vi "getParameters.vi"(11 "AbortLowerM1M3Command in":refnum<class "AbortLowerM1M3Command.lvclass">) -> (2 "Parameters":T1, 3 "AbortLowerM1M3Command out":refnum<class "AbortLowerM1M3Command.lvclass">)   [LabVIEW 2016, in "AbortLowerM1M3Command.lvclass"]
uses:
  AbortLowerM1M3Command.lvclass
  DataTypes/Topics/CommandAbortLowerM1M3.ctl
  DataTypes/Topics/Parts/CommandId.ctl
  AbortLowerM1M3Command.lvclass/AbortLowerM1M3Command.ctl
  DataTypes/Topics/M1M3SupportTopics.lvlib
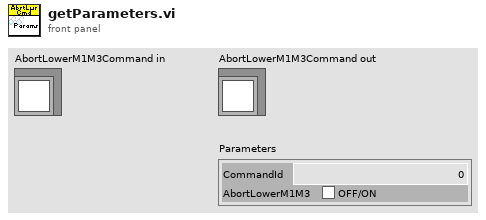
[diagram p1: front panel]
types:
  T1 = typedef "M1M3SupportTopics.lvlib/CommandAbortLowerM1M3.ctl" = cluster{"CommandId":T2, "AbortLowerM1M3":bool}
  T2 = typedef "M1M3SupportTopics.lvlib/CommandId.ctl" = i32
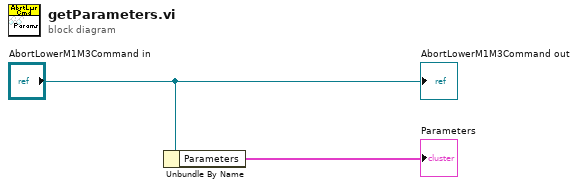
[diagram p0: block diagram]
diagram:
  n1 = Unbundle By Name("AbortLowerM1M3Command in") -> ("Parameters"=→"Parameters":T1)
  "AbortLowerM1M3Command out" <- "AbortLowerM1M3Command in"
